vi "ATF-Pump-DI FGV.vi"(8 "error in":errorcluster, 9 "DI Seq  IN":T1(array[cluster]), 11 "Enum":enum16{"Read", "Write "}(ring)) -> (0 "error out":errorcluster, 1 "DI Seq  OUT":T1(array[cluster]))   [LabVIEW 2022 SP3]
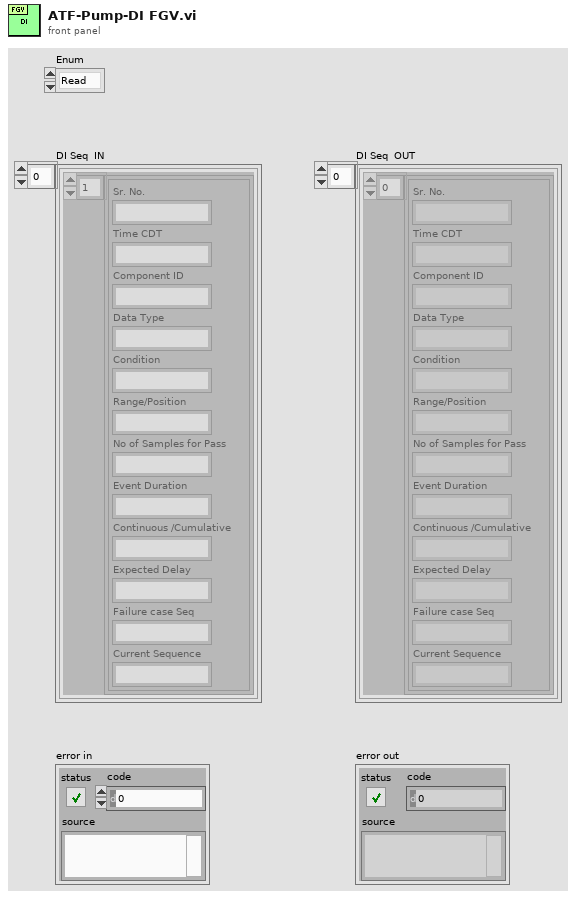
[diagram p1: front panel]
types:
  T1 = cluster{cluster{"Sr. No.":string, "Time CDT":string, "Component ID":string, "Data Type":string, "Condition":string, "Range/Position":string, "No of Samples for Pass":string, "Event Duration":string, "Continuous /Cumulative":string, "Expected Delay":string, "Failure case Seq":string, "Current Sequence":string}[]}[]
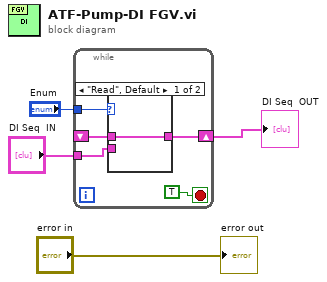
[diagram p0: block diagram]
diagram:
  n1 = while {
    tunnel: "Enum" -> [w9]
    tunnel: "DI Seq  IN" -> [w7]
    shift-right: [w6] -> w1
    shift-left: _ -> [w5]
    stop <- TRUE stop-if-true
    n2 = case shown="\"Read\", Default" w9 {
      tunnel: w7 -> [_ w11]
      tunnel: [w10 w11] -> w6
      tunnel: w5 -> [w10 _]
      frame "Read", Default {
      }
      frame "Write " {
      }
    }
  }
  "DI Seq  OUT" <- w1
  "error out" <- "error in"
